vi "SplitAppended.vi"(9 "Appended errors in":errorcluster) -> (1 "Errors out":errorcluster[](array[cluster]))   [LabVIEW 2017, in "GPError.lvlib"]
doc: "Splits <B>Appended errors in</B> up into an array of individual <B>Errors out</B>.\n\nThis VI is inlined.\n\nSteen Schmidt\nGPower\n15/7 2013"
uses:
  GPError.lvlib
panel:
  # "Copyright © 2014\nGPower\nSee enclosed license file for terms and conditions"
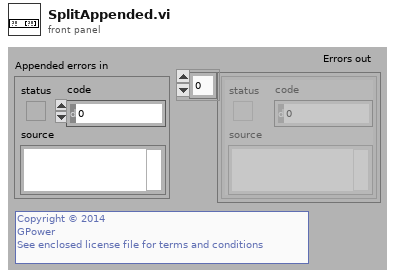
[diagram p1: front panel]
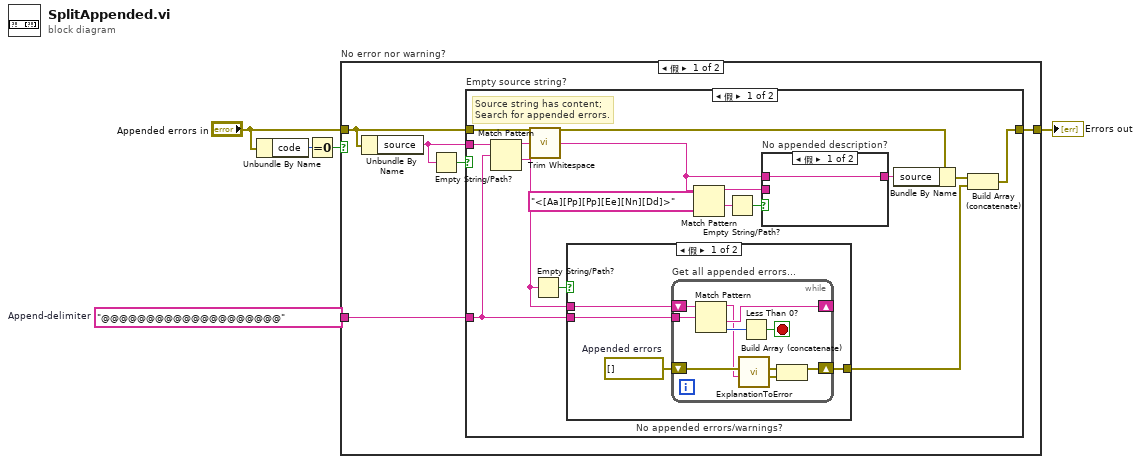
[diagram p0: block diagram]
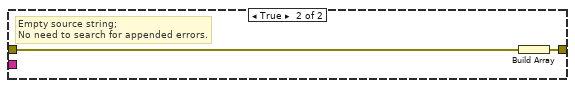
[diagram p4: hidden frame]
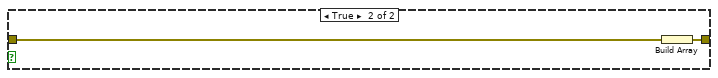
[diagram p5: hidden frame]
diagram:
  w2 = "@@@@@@@@@@@@@@@@@@@@"  # Append-delimiter
  n1 = Unbundle By Name("Appended errors in") -> ("code"=w3:i32)
  n2 = Equal To 0?(x=w3) -> (x = 0?=w1:bool)
  n3 = case "No error nor warning?" shown="假" w1 {
    tunnel: [w10 w43] -> w5
    tunnel: "Appended errors in" -> [w9 w44]
    tunnel: w2 -> [w8 _]
    frame False {
      n4 = Unbundle By Name(w9) -> ("source"=w7:string)
      n5 = Empty String/Path?(string/path=w7) -> (empty?=w6:bool)
      n6 = case "Empty source string?" shown="假" w6 {
        tunnel: w7 -> [w25 _]
        tunnel: [w22 w41] -> w10
        tunnel: w9 -> [w12 w42]
        tunnel: w8 -> [w11 _]
        frame False {
          # "Source string has content;\nSearch for appended errors."
          n7 = Match Pattern(string=w25, regular expression=w11) -> (before substring=w24:string, after substring=w13:string)  [unwired: 1 in, 2 out]
          n8 = call <vilib>:"Trim Whitespace.vi"("string"=w24) -> ("trimmed string"=w17:string)  [unwired: 1 in]
          n9 = Empty String/Path?(string/path=w13) -> (empty?=w14:bool)
          n10 = case "No appended errors/warnings?" shown="假" w14 {
            tunnel: w13 -> [w29 _]
            tunnel: w11 -> [w28 _]
            tunnel: [w26 _] -> w15
            frame False {
              w27 = errorcluster[] []  # Appended errors
              n11 = while "Get all appended errors..." {
                shift-right: [w32] -> _
                shift-left: w29 -> [w38]
                tunnel: w28 -> [w37]
                shift-right: [w33] -> w26
                shift-left: w27 -> [w35]
                stop <- w34 stop-if-true
                n12 = Match Pattern(string=w38, regular expression=w37) -> (before substring=w31:string, after substring=w32:string, offset past match=w36:i32)  [unwired: 1 in, 1 out]
                n13 = call "ExplanationToError.vi"("Explanation in"=w31) -> ("Error out"=w30:errorcluster)  [unwired: 10 in]
                n14 = Less Than 0?(x=w36) -> (x < 0?=w34:bool)
                n15 = Build Array (concatenate)(w35, w30) -> (w33:errorcluster[])
              }
            }
            frame True {
            }
          }
          n16 = Match Pattern(string=w17, regular expression="<[Aa][Pp][Pp][Ee][Nn][Dd]>") -> (before substring=w18:string, after substring=w20:string)  [unwired: 1 in, 2 out]
          n17 = Empty String/Path?(string/path=w20) -> (empty?=w19:bool)
          n18 = case "No appended description?" shown="假" w19 {
            tunnel: w18 -> [_ w40]
            tunnel: w17 -> [w39 _]
            tunnel: [w39 w40] -> w16
            frame False {
            }
            frame True {
            }
          }
          n19 = Bundle By Name(cluster=w12, "source"=w16) -> (w23:errorcluster)
          n20 = Build Array (concatenate)(w23, w15) -> (w22:errorcluster[])
        }
        frame True {
          # "Empty source string;\nNo need to search for appended errors."
          n21 = Build Array(w42) -> (w41:errorcluster[])
        }
      }
    }
    frame True {
      n22 = Build Array(w44) -> (w43:errorcluster[])
    }
  }
  "Errors out" <- w5
